vi "Merge Error Ex.vi"(7 "Is error? (False)":bool, 10 "main error in (no error)":errorcluster, 11 "second error in":errorcluster) -> (2 "error out":errorcluster)   [LabVIEW 2020]
doc: "This VI will merge two errors but only if 'Is error?' is true. Note that merging means only the first nonempty error will be at the output. In this VI main input error has preference."
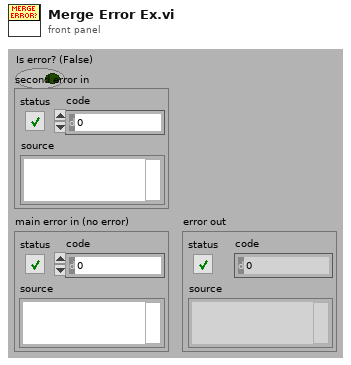
[diagram p1: front panel]
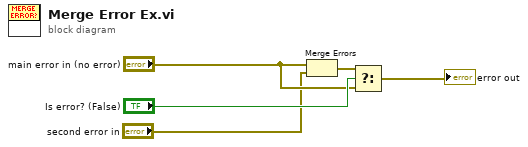
[diagram p0: block diagram]
diagram:
  n1 = Merge Errors("main error in (no error)", "second error in") -> (w5:errorcluster)
  n2 = Select(t=w5, s="Is error? (False)", f="main error in (no error)") -> (s? t:f=→"error out":errorcluster)
